vi "hw5_1.vi"() -> ()   [LabVIEW 2014]
panel:
  out "samples per acquisition 2":dbl=10000.0
  out "sampling rate (samples/sec) 2":dbl=1000.0
  out "Pass":bool
  in  "stop":bool
  in  "Menu Cluster":T1
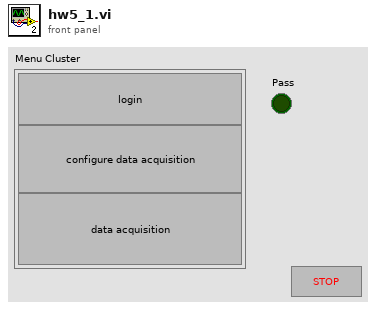
[diagram p1: front panel]
types:
  T1 = cluster{"login":bool, "configure":bool, "acquire data":bool}
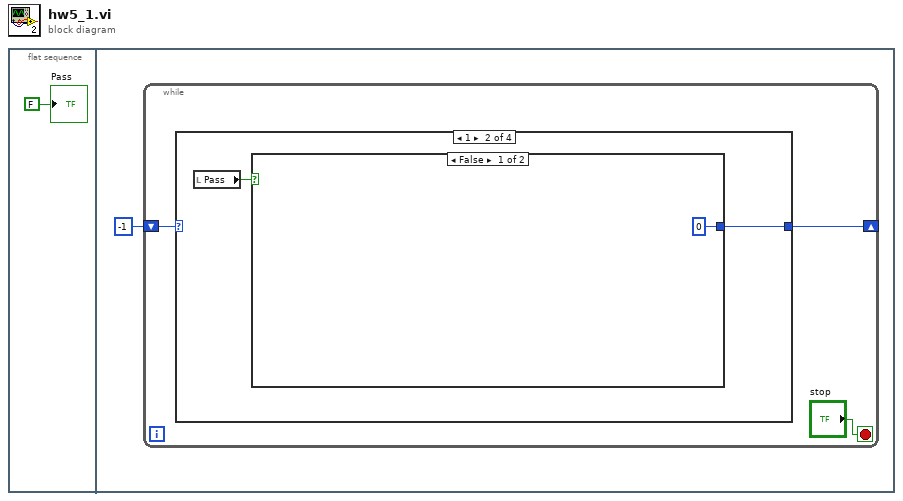
[diagram p0: block diagram]
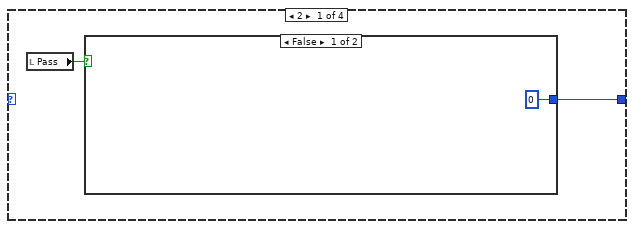
[diagram p2: hidden frame]
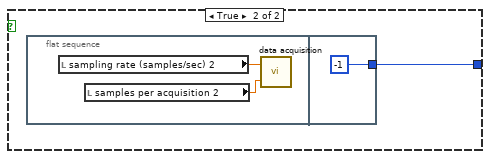
[diagram p3: hidden frame]
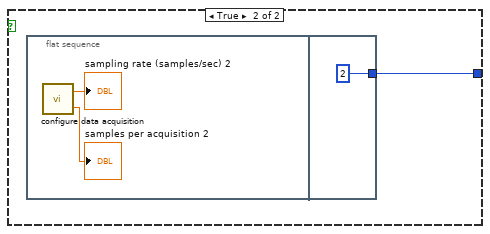
[diagram p4: hidden frame]
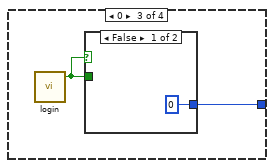
[diagram p5: hidden frame]
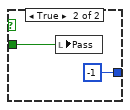
[diagram p6: hidden frame]
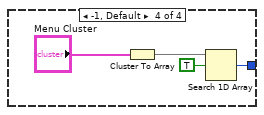
[diagram p7: hidden frame]
diagram:
  n1 = flat-sequence {
    frame #0 {
      "Pass" <- FALSE ("Pass")
    }
    frame #1 {
      n2 = while {
        shift-right: [w3] -> _
        shift-left: -1 -> [w4]
        stop <- "stop" stop-if-true
        n3 = case shown="1" w4 {
          tunnel: [w7 w13 w21 w26] -> w3
          frame 2 {
            n4 = local read "Pass"() -> (w6:bool)
            n5 = case shown="False" w6 {
              tunnel: [0 w9] -> w7
              frame False {
              }
              frame True {
                n6 = flat-sequence {
                  tunnel: [-1] -> w9
                  frame #0 {
                    n7 = local read "sampling rate (samples/sec) 2"() -> (w11:dbl)
                    n8 = local read "samples per acquisition 2"() -> (w10:dbl)
                    n9 = call "data acquisition.vi"("samples per acquisition"=w10, "samples rate"=w11) -> ()  [unwired: 1 in]
                  }
                  frame #1 {
                  }
                }
              }
            }
          }
          frame 1 {
            n10 = local read "Pass"() -> (w14:bool)
            n11 = case shown="False" w14 {
              tunnel: [0 w16] -> w13
              frame False {
              }
              frame True {
                n12 = flat-sequence {
                  tunnel: [2] -> w16
                  frame #0 {
                    n13 = call "configure data acquisition.vi"() -> ("sampling rate (samples/sec) 2"=→"sampling rate (samples/sec) 2":dbl, "samples per acquisition 2"=→"samples per acquisition 2":dbl)  [unwired: 1 in]
                  }
                  frame #1 {
                  }
                }
              }
            }
          }
          frame 0 {
            n14 = call "login.vi"() -> ("Pass"=w20:bool)  [unwired: 1 in, 2 out]
            n15 = case shown="False" w20 {
              tunnel: [0 -1] -> w21
              tunnel: w20 -> [_ w23]
              frame False {
              }
              frame True {
                n16 = local write "Pass"(w23) -> ()
              }
            }
          }
          frame -1, Default {
            n17 = Cluster To Array(cluster="Menu Cluster") -> (array=w28:bool[])
            n18 = Search 1D Array(1D array=w28, element=TRUE) -> (index of element=w26:i32)  [unwired: 1 in]
          }
        }
      }
    }
  }
